vi "Perf_Measure_Gen_Noisy_Img-1.vi"() -> ()   [LabVIEW 2020]
panel:
  in  "Constant \nGeneration":bool
  in  "Single Cores \nSubprograms":enum16{"1", "2"}(ring)
  out "ms for U16 pixels\nto img transfer":u32
  out "Image":T1(plugin-control)
  in  "stop":bool
  in  "Generate Pic":bool
  out "Raw Pixel Values":u16[][](graph)
  out "ms for generation\nof single noisy img":u32
  in  "Width":i32=2 min=2 max=10000 step=1
  in  "Height":i32=2 min=2 max=5000 step=1
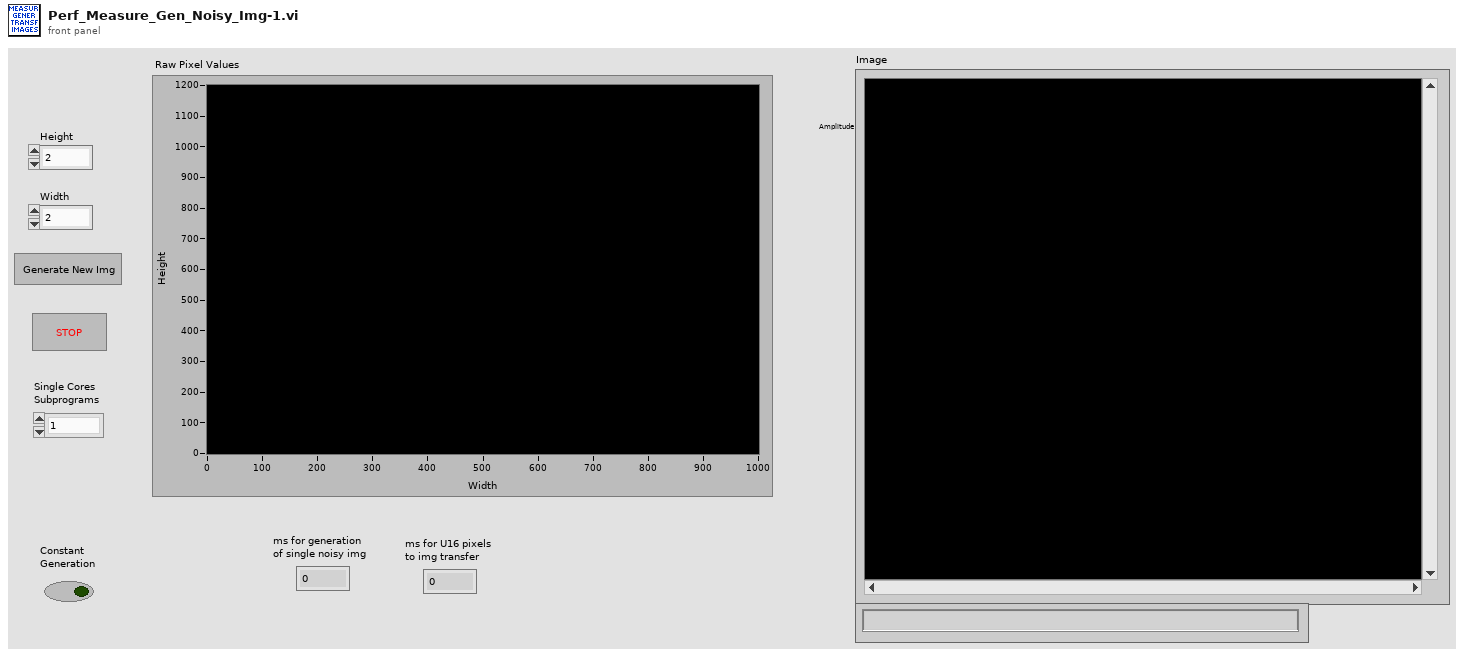
[diagram p1: front panel]
types:
  T1 = typedef "IMAQ Image.ctl" = refnum<image>
  T2 = typedef "Image Type" = u32
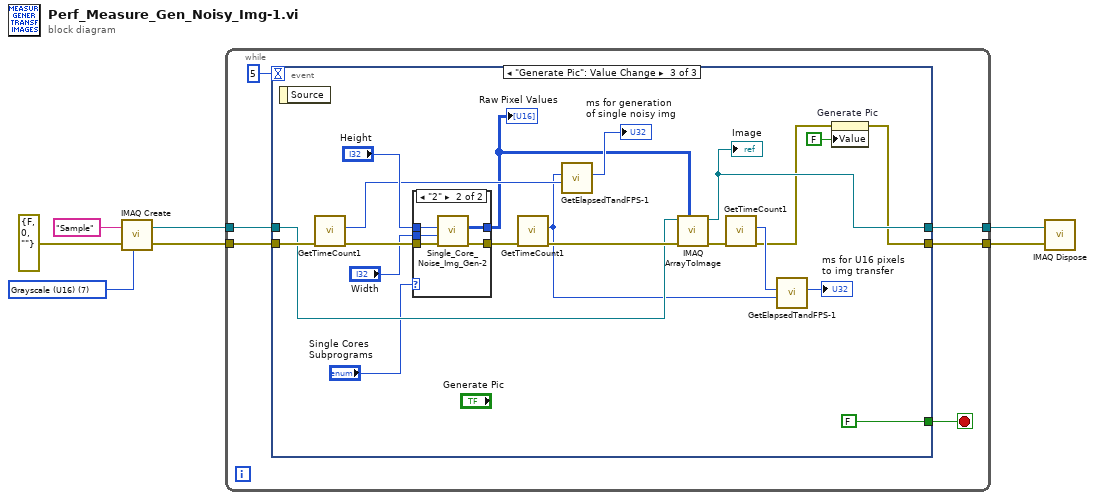
[diagram p0: block diagram]
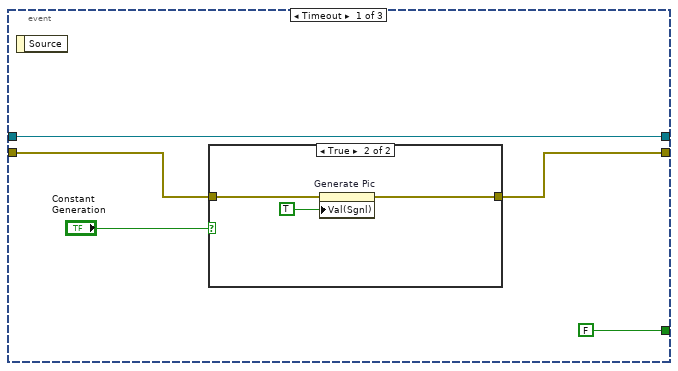
[diagram p2: hidden frame]
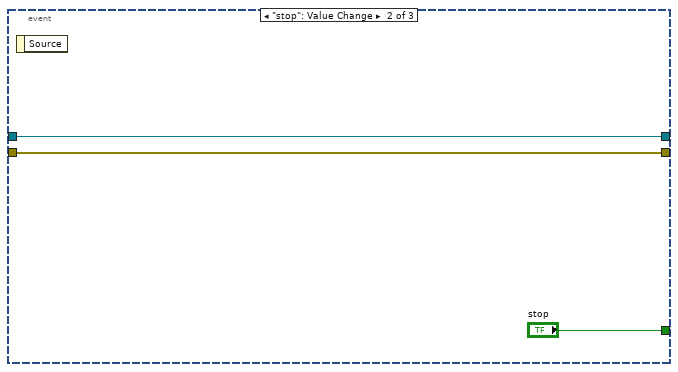
[diagram p4: hidden frame]
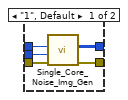
[diagram p5: hidden frame]
diagram:
  w5 = T2 7 items=["Grayscale (U8)", "Grayscale (I16)", "Grayscale (SGL)", "Complex (CSG)", "RGB (U32)", "HSL (U32)", "RGB (U64)", "Grayscale (U16)"] ("Image Type")
  n1 = call "IMAQ Create"("Image Name"="Sample", "Image Type"=w5, "error in (no error)"=errorcluster {"status"=FALSE, "code"=0, "source"=""}) -> ("New Image"=w2:T1, "error out"=w4:errorcluster)  [unwired: 2 in]
  n2 = while {
    tunnel: w4 -> [w13]
    tunnel: [w12] -> w3
    tunnel: w2 -> [w11]
    tunnel: [w10] -> w1
    stop <- w9 stop-if-true
    n3 = event shown="[2] \"Generate Pic\": Value Change" {
      selector: _ -> [_ _ _]
      dyn-events: _ -> [_ _ _]
      timeout: 5 -> [_ _ _]
      tunnel: w13 -> [w15 w24 w38]
      tunnel: [w14 w24 w27] -> w12
      tunnel: w11 -> [w18 w23 w36]
      tunnel: [w18 w23 w33] -> w10
      tunnel: [FALSE ("stop") "stop" FALSE ("stop")] -> w9
      event Timeout {
        n4 = event-data() -> ()  [unwired: 1 in, 1 out]
        n5 = case shown="True" "Constant \nGeneration" {
          tunnel: w15 -> [w19 w22]
          tunnel: [w19 w21] -> w14
          frame False {
          }
          frame True {
            n6 = property on="Generate Pic" class="Bool (strict)"(error in=w22, "Val(Sgnl)"=TRUE ("Value (Signaling)")) -> (error out=w21:errorcluster)  [unwired: 1 in, 1 out]
          }
        }
      }
      event "stop": Value Change {
        n7 = event-data() -> ()  [unwired: 1 in, 1 out]
      }
      event "Generate Pic": Value Change {
        n8 = event-data() -> ()  [unwired: 1 in, 1 out]
        n9 = call "GetTimeCount1.vi"("error IN"=w38) -> ("error OUT"=w44:errorcluster, "[OUT] Timer Count"=w41:u32)  [unwired: 9 in]
        n10 = case shown="\"2\"" "Single Cores \nSubprograms" {
          tunnel: w44 -> [w50 w55]
          tunnel: "Height" -> [w49 w53]
          tunnel: [w48 w52] -> w42
          tunnel: "Width" -> [w47 w54]
          tunnel: [w46 w51] -> w35
          frame "1", Default {
            n11 = call "Single_Core_Noise_Img_Gen.vi"("error IN"=w50, "[IN] Width"=w47, "[IN] Height"=w49) -> ("error OUT"=w48:errorcluster, "[OUT] U16 Pixel Img"=w46:u16[][])  [unwired: 7 in]
          }
          frame "2" {
            n12 = call "Single_Core_Noise_Img_Gen-2.vi"("error IN"=w55, "[IN] Width"=w54, "[IN] Height"=w53) -> ("error OUT"=w52:errorcluster, "[OUT] U16 Pixel Img"=w51:u16[][])  [unwired: 7 in]
          }
        }
        "Raw Pixel Values" <- w35
        n13 = call "GetTimeCount1.vi"("error IN"=w42) -> ("error OUT"=w37:errorcluster, "[OUT] Timer Count"=w31:u32)  [unwired: 9 in]
        n14 = call "GetElapsedTandFPS-1.vi"("[IN] Timer Count Before ALL [ms]"=w41, "[IN] Timer Count After ALL [ms]"=w31) -> ("[OUT] Elapsed time [ms]"=→"ms for generation\nof single noisy img":u32)  [unwired: 3 in, 2 out]
        n15 = call "IMAQ ArrayToImage"("Image Pixels (U16)"=w35, "error in (no error)"=w37, "Image"=w36) -> ("error out"=w34:errorcluster, "Image Out"=w33:T1)  [unwired: 7 in]
        "Image" <- w33
        n16 = call "GetTimeCount1.vi"("error IN"=w34) -> ("error OUT"=w28:errorcluster, "[OUT] Timer Count"=w32:u32)  [unwired: 9 in]
        n17 = call "GetElapsedTandFPS-1.vi"("[IN] Timer Count Before ALL [ms]"=w31, "[IN] Timer Count After ALL [ms]"=w32) -> ("[OUT] Elapsed time [ms]"=→"ms for U16 pixels\nto img transfer":u32)  [unwired: 3 in, 2 out]
        n18 = property on="Generate Pic" class="Bool (strict)"(error in=w28, "Value"=FALSE ("Generate Pic")) -> (error out=w27:errorcluster)  [unwired: 1 in, 1 out]
      }
    }
  }
  n19 = call "IMAQ Dispose"("Image"=w1, "error in (no error)"=w3) -> ()  [unwired: 4 in, 1 out]
